vi "Quiz4_TP059851_Sim Yoke Shin_Server.vi"() -> ()   [LabVIEW 2020]
panel:
  out "Blinking Warning":bool
  # "Server"
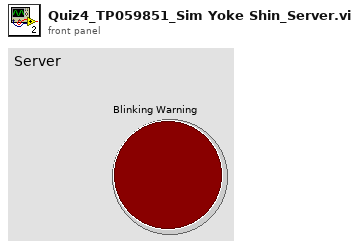
[diagram p1: front panel]
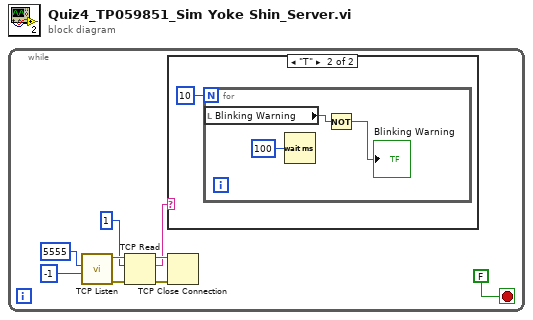
[diagram p0: block diagram]
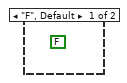
[diagram p2: hidden frame]
diagram:
  n1 = while {
    stop <- FALSE stop-if-true
    n2 = call <vilib>:"TCP Listen.vi"("timeout ms (wait forever: -1)"=-1, "port"=u16 5555) -> ("error out"=w2:errorcluster, "connection ID"=w3:refnum<k5>)  [unwired: 5 in, 3 out]
    n3 = TCP Read(connection ID=w3, bytes to read=1, error in (no error)=w2) -> (connection ID out=w9:refnum<k5>, data out=w5:string, error out=w8:errorcluster)  [unwired: 2 in]
    n4 = case shown="\"T\"" w5 {
      frame "F", Default {
        (unwired) FALSE
      }
      frame "T" {
        n5 = for {
          N: 10 -> [_]
          n6 = local read "Blinking Warning"() -> (w13:bool)
          n7 = Wait (ms)(milliseconds to wait=u32 100) -> ()  [unwired: 1 out]
          n8 = Not(x=w13) -> (.not. x?=→"Blinking Warning":bool)
        }
      }
    }
    n9 = TCP Close Connection(connection ID=w9, error in (no error)=w8) -> ()  [unwired: 1 in, 2 out]
  }
